vi "Queue Caller.vi"(9 "Priority?":bool, 10 "Msg Strategy":refnum<class "Msg Strategy.lvclass">, 11 "Base Queue jettl in":refnum<class "Base Queue jettl.lvclass">) -> (3 "Base Queue jettl out":refnum<class "Base Queue jettl.lvclass">)   [LabVIEW 2021, in "jettl.lvlib" / "Base Queue jettl.lvlib" / "Base Queue jettl.lvclass"]
uses:
  Base Queue jettl.lvclass
  Msg Strategy/Msg Strategy.lvclass
  Base Queue jettl.lvclass/Base Queue jettl.ctl
  jettl.lvlib
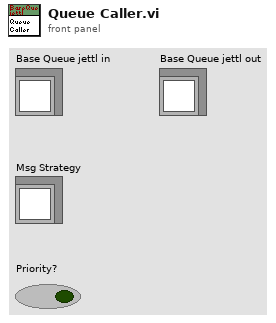
[diagram p1: front panel]
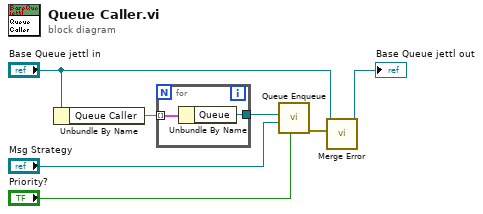
[diagram p0: block diagram]
diagram:
  n1 = Unbundle By Name("Base Queue jettl in") -> ("Queue Caller"=w2:map{string, refnum<data-value>})
  n2 = for {
    tunnel: [w8] -> w1
    tunnel: w2 -> [w9] mode=indexing
    n3 = Unbundle By Name(w9) -> ("Queue"=w8:refnum<data-value>)
  }
  n4 = call "Queue Enqueue.vi"("Priority?"="Priority?", "Msg Strategy"="Msg Strategy", "Queue"=w1) -> ("error out"=w3:errorcluster)  [unwired: 8 in]
  n5 = call-dynamic "Merge Error.vi"("Error"=w3, "Base Queue jettl in"="Base Queue jettl in") -> ("Base Queue jettl out"=→"Base Queue jettl out":refnum<class "Base Queue jettl.lvclass">)  [unwired: 9 in]
